vi "Terminal-ModbusEthernet-ReadWriteRegisters.vi"(6 "error in":errorcluster, 7 "write operation timeout (ms)":i32=5000 caption="写操作超时（毫秒）", 8 "read operation timeout (ms)":i32=5000 caption="读操作超时（毫秒）", 9 "Modbus data":cluster{"Data":variant, "State":string}) -> (0 "error out":errorcluster, 3 "register values":u16[](array[numeric]) caption="寄存器值")   [LabVIEW 2014]
uses:
  <vilib>/Modbus/subvis/Modbus API/Modbus API.lvclass/Modbus API.ctl
  <vilib>/Modbus/subvis/Transmission Data Unit (ADU)/Transmission Data Unit/Transmission Data Unit.lvclass/Transmission Data Unit.ctl
  <vilib>/Modbus/master/Data Access/Unit ID/Set Unit ID Property.vi
  <vilib>/Modbus/subvis/Transmission Data Unit (ADU)/Transmission Data Unit/Data Access/Unit ID/Write Unit ID.vi
  <vilib>/Modbus/subvis/Modbus API/Read Transmission Data Unit.vi
  <vilib>/Modbus/subvis/Modbus API/Write Transmission Data Unit.vi
  <vilib>/Modbus/master/Create Master Instance (TCP).vi
  <vilib>/Modbus/subvis/Transmission Data Unit (ADU)/Transmission Data Unit/Transmission Data Unit.lvclass
  <vilib>/Modbus/master/Modbus Master.lvclass
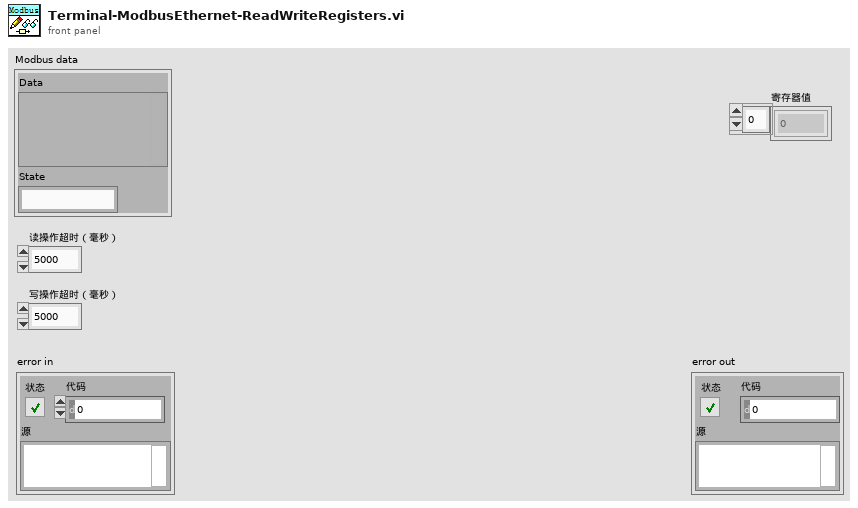
[diagram p1: front panel]
types:
  T1 = cluster{"Unit ID":u8, "Starting Address":u16, "Quantity":u16}
  T2 = cluster{"Unit ID":u8, "Address":u16, "Register":u16}
  T3 = cluster{"Unit ID":u8, "Starting Address":u16, "Registers":u16[]}
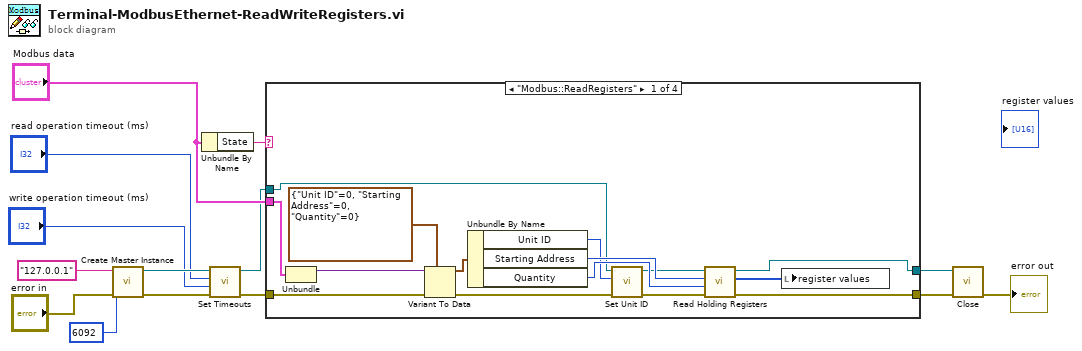
[diagram p0: block diagram]
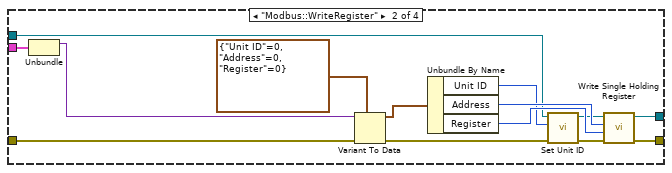
[diagram p2: hidden frame]
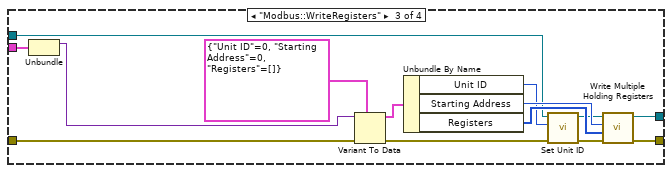
[diagram p3: hidden frame]
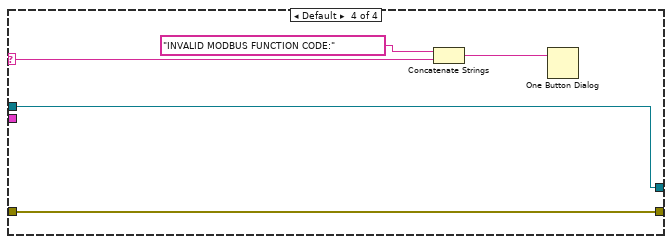
[diagram p4: hidden frame]
diagram:
  n1 = call-poly <vilib>:"Create Master Instance.vi"("error in (no error)"="error in", "port (502)"=u16 6092, "address"="127.0.0.1" ("地址")) -> ("error out"=w8:errorcluster, "TCP master instance"=w7:refnum<class "Modbus Master.lvclass">)  [unwired: 7 in]
  n2 = Unbundle By Name("Modbus data") -> ("State"=w14:string)
  n3 = call <vilib>:"Set Timeouts.vi"("error in (no error)"=w8, "write operation timeout (ms)"="write operation timeout (ms)", "read operation timeout (ms)"="read operation timeout (ms)", "Modbus master in"=w7) -> ("error out"=w9:errorcluster, "Modbus master out"=w10:refnum<class "Modbus Master.lvclass">)  [unwired: 6 in]
  n4 = case shown="\"Modbus::ReadRegisters\"" w14 {
    selector: w14 -> [_ _ _ w60]
    tunnel: "Modbus data" -> [w29 w42 w54 _]
    tunnel: w9 -> [w26 w43 w53 w58]
    tunnel: w10 -> [w17 w31 w45 w59]
    tunnel: [w24 w38 w52 w59] -> w4
    tunnel: [w23 w35 w49 w58] -> w3
    frame "Modbus::ReadRegisters" {
      n5 = Unbundle(w29) -> ("Data"=w28:variant)  [unwired: 1 out]
      n6 = Variant To Data(error in=w26, type=T1 {"Unit ID"=0, "Starting Address"=0, "Quantity"=0}, Variant=w28) -> (data=w27:T1, error out=w20:errorcluster)
      n7 = Unbundle By Name(w27) -> ("Unit ID"=w16:u8, "Starting Address"=w22:u16, "Quantity"=w21:u16)
      n8 = call <vilib>:"Set Unit ID.vi"("error in (no error)"=w20, "unit ID"=w16, "Modbus master in"=w17) -> ("error out"=w19:errorcluster, "Modbus master out"=w18:refnum<class "Modbus Master.lvclass">)  [unwired: 7 in]
      n9 = call-dynamic "Read Holding Registers.vi"("error in (no error)"=w19, "number of holding registers"=w21, "starting address"=w22, "Modbus master in"=w18) -> ("error out"=w23:errorcluster, "register values"=w15:u16[], "Modbus master out"=w24:refnum<class "Modbus Master.lvclass">)  [unwired: 5 in]
      n10 = local write "register values"(w15) -> ()
    }
    frame "Modbus::WriteRegister" {
      n11 = Unbundle(w42) -> ("Data"=w41:variant)  [unwired: 1 out]
      n12 = Variant To Data(error in=w43, type=T2 {"Unit ID"=0, "Address"=0, "Register"=0}, Variant=w41) -> (data=w39:T2, error out=w33:errorcluster)
      n13 = Unbundle By Name(w39) -> ("Unit ID"=w32:u8, "Address"=w37:u16, "Register"=w36:u16)
      n14 = call <vilib>:"Set Unit ID.vi"("error in (no error)"=w33, "unit ID"=w32, "Modbus master in"=w31) -> ("error out"=w34:errorcluster, "Modbus master out"=w30:refnum<class "Modbus Master.lvclass">)  [unwired: 7 in]
      n15 = call-dynamic "Write Single Holding Register.vi"("error in (no error)"=w34, "holding register value"=w36, "address"=w37, "Modbus master in"=w30) -> ("error out"=w35:errorcluster, "Modbus master out"=w38:refnum<class "Modbus Master.lvclass">)  [unwired: 6 in]
    }
    frame "Modbus::WriteRegisters" {
      n16 = Unbundle(w54) -> ("Data"=w57:variant)  [unwired: 1 out]
      n17 = Variant To Data(error in=w53, type=T3 {"Unit ID"=0, "Starting Address"=0, "Registers"=[]}, Variant=w57) -> (data=w55:T3, error out=w47:errorcluster)
      n18 = Unbundle By Name(w55) -> ("Unit ID"=w46:u8, "Starting Address"=w51:u16, "Registers"=w50:u16[])
      n19 = call <vilib>:"Set Unit ID.vi"("error in (no error)"=w47, "unit ID"=w46, "Modbus master in"=w45) -> ("error out"=w48:errorcluster, "Modbus master out"=w44:refnum<class "Modbus Master.lvclass">)  [unwired: 7 in]
      n20 = call-dynamic "Write Multiple Holding Registers.vi"("error in (no error)"=w48, "holding register values"=w50, "starting address"=w51, "Modbus master in"=w44) -> ("error out"=w49:errorcluster, "Modbus master out"=w52:refnum<class "Modbus Master.lvclass">)  [unwired: 6 in]
    }
    frame Default {
      n21 = Concatenate Strings("INVALID MODBUS FUNCTION CODE:", w60) -> (w61:string)
      n22 = One Button Dialog(message=w61) -> ()  [unwired: 1 in, 1 out]
    }
  }
  n23 = call-dynamic "Close.vi"("error in (no error)"=w3, "Modbus master in"=w4) -> ("error out"=→"error out":errorcluster)  [unwired: 9 in]
